vi "SaveToTblHist.vi"(8 "error in (no error)":errorcluster, 10 "OldTable (reset)":string[][](table), 11 "Table History ref":refnum<vi>) -> (0 "error out":errorcluster)   [LabVIEW 2013]
doc: "Add OldTable to the referred Table Undo (history) array. If TableHistory ref is not wired, no history is saved and currently there is no warning! CAUTION: Empty 'OldTable' signals that the history should be reset! This will be used for changes that cannot be undone like adding/removing devices. The default for OldTable is empty, causing it to reset if unwired."
uses:
  TypeDefs/TableHistory.ctl
  TypeDefs/TableArray.ctl
panel:
  out "Invalid ref?":bool
  out "reset?":bool
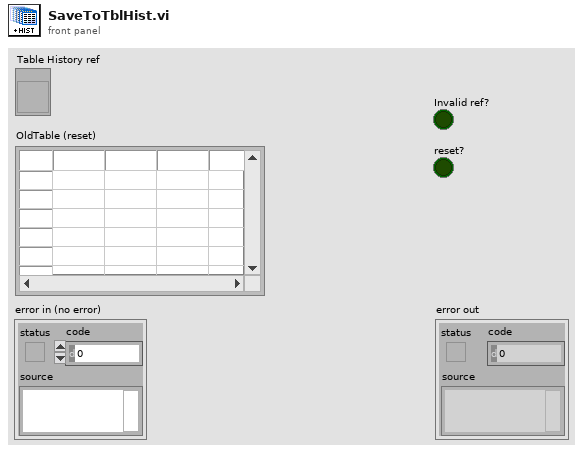
[diagram p1: front panel]
types:
  T1 = typedef "TableHistory.ctl" = cluster{"OldTable Array":T2, "Undo pointer":i32}
  T2 = typedef "TableArray.ctl" = cluster{"OldTable":string[][]}[]
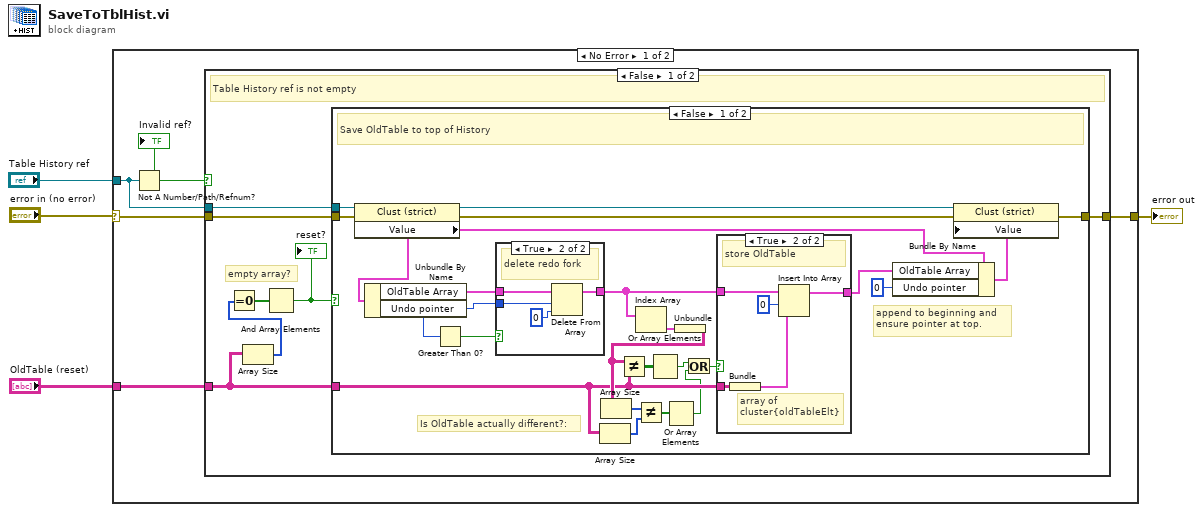
[diagram p0: block diagram]
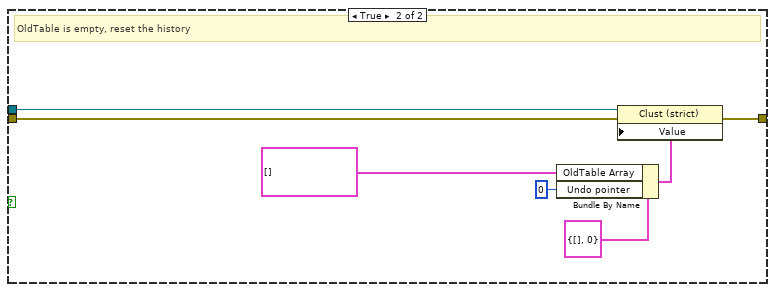
[diagram p4: hidden frame]
diagram:
  n1 = case shown="No Error" "error in (no error)" {
    selector: "error in (no error)" -> [w9 w59]
    tunnel: [w8 w59] -> w3
    tunnel: "OldTable (reset)" -> [w7 _]
    tunnel: "Table History ref" -> [w6 _]
    frame No Error {
      n2 = Not A Number/Path/Refnum?(number/path/refnum=w6) -> (NaN/Path/Refnum?=w5:bool)
      "Invalid ref?" <- w5
      n3 = case shown="False" w5 {
        tunnel: w9 -> [w13 w58]
        tunnel: [w12 w58] -> w8
        tunnel: w7 -> [w11 _]
        tunnel: w6 -> [w10 _]
        frame False {
          # "empty array?"
          # "Table History ref is not empty"
          n4 = Array Size(array=w11) -> (size(s)=w15:i32[])
          n5 = Equal To 0?(x=w15) -> (x = 0?=w16:bool[])
          n6 = And Array Elements(Boolean array=w16) -> (logical AND=w14:bool)
          "reset?" <- w14
          n7 = case shown="False" w14 {
            tunnel: w13 -> [w39 w56]
            tunnel: [w32 w55] -> w12
            tunnel: w10 -> [w38 w54]
            tunnel: w11 -> [w20 _]
            frame False {
              # "Is OldTable actually different?:"
              # "append to beginning and\nensure pointer at top."
              # "Save OldTable to top of History"
              n8 = property class="Clust (strict)"(reference=w38, error in=w39) -> (reference out=w34:refnum<vi>, error out=w33:errorcluster, "Value"=w31:T1)
              n9 = Unbundle By Name(w31) -> ("OldTable Array"=w37:T2, "Undo pointer"=w36:i32)
              n10 = Greater Than 0?(x=w36) -> (x > 0?=w35:bool)
              n11 = case shown="True" w35 {
                tunnel: w37 -> [w46 w50]
                tunnel: w36 -> [_ w49]
                tunnel: [w46 w47] -> w27
                frame False {
                  # "none for redo"
                }
                frame True {
                  # "delete redo fork"
                  n12 = Delete From Array(array=w50, length=w49, index=0) -> (array with subset deleted=w47:T2)  [unwired: 1 out]
                }
              }
              n13 = Array Size(array=w20) -> (size(s)=w21:i32[])
              n14 = Index Array(array=w27) -> (element=w26:cluster{"OldTable":string[][]})  [unwired: 1 in]
              n15 = Unbundle(w26) -> ("OldTable"=w22:string[][])
              n16 = Array Size(array=w22) -> (size(s)=w23:i32[])
              n17 = Not Equal?(x=w22, y=w20) -> (x != y?=w25:bool[][])
              n18 = Not Equal?(x=w23, y=w21) -> (x != y?=w18:bool[])
              n19 = Or Array Elements(Boolean array=w25) -> (logical OR=w17:bool)
              n20 = Or Array Elements(Boolean array=w18) -> (logical OR=w19:bool)
              n21 = Or(x=w17, y=w19) -> (x .or. y?=w24:bool)
              n22 = case shown="True" w24 {
                tunnel: [w40 w45] -> w29
                tunnel: w27 -> [w40 w43]
                tunnel: w20 -> [_ w41]
                frame False {
                  # "already saved!"
                }
                frame True {
                  # "array of \ncluster{oldTableElt}"
                  # "store OldTable"
                  n23 = Bundle("OldTable (reset)"=w41) -> (w42:cluster{"OldTable (reset)":string[][]})  [unwired: 1 in]
                  n24 = Insert Into Array "Insert Into Array"(array=w43, index=0, new element=w42) -> (w45:T2)
                }
              }
              n25 = Bundle By Name(cluster=w31, "OldTable Array"=w29, "Undo pointer"=0) -> (w30:T1)
              n26 = property class="Clust (strict)"(reference=w34, error in=w33, "Value"=w30) -> (error out=w32:errorcluster)  [unwired: 1 out]
            }
            frame True {
              # "OldTable is empty, reset the history"
              n27 = Bundle By Name(cluster=T1 {"OldTable Array"=[], "Undo pointer"=0} ("Value"), "OldTable Array"=T2 [], "Undo pointer"=0) -> (w57:T1)
              n28 = property class="Clust (strict)"(reference=w54, error in=w56, "Value"=w57) -> (error out=w55:errorcluster)  [unwired: 1 out]
            }
          }
        }
        frame True {
          # "possibly warn user here"
          # "no refnum to Table history (do nothing)"
        }
      }
    }
    frame Error {
    }
  }
  "error out" <- w3
